vi "Filter new tree data.vi"(7 "Headers":string[](array[string]), 8 "error in":errorcluster, 9 "Root row":string[](array[string]), 10 "Child rows":string[][](array[string]), 11 "Filter":refnum<vi>) -> (0 "error out":errorcluster, 2 "Filtered child rows":string[][](array[string]), 3 "Filtered root row":string[](array[string]))   [LabVIEW 2025, in "CAN-LIN Raw Bus Capture UI.lvlib"]
uses:
  CAN-LIN Raw Bus Capture UI.lvlib
  <vilib>/Utility/error.llb/whitespace.ctl
  <vilib>/Utility/error.llb/Trim Whitespace One-Sided.vi
  Table_Filtering/Table_Filtering.lvlib
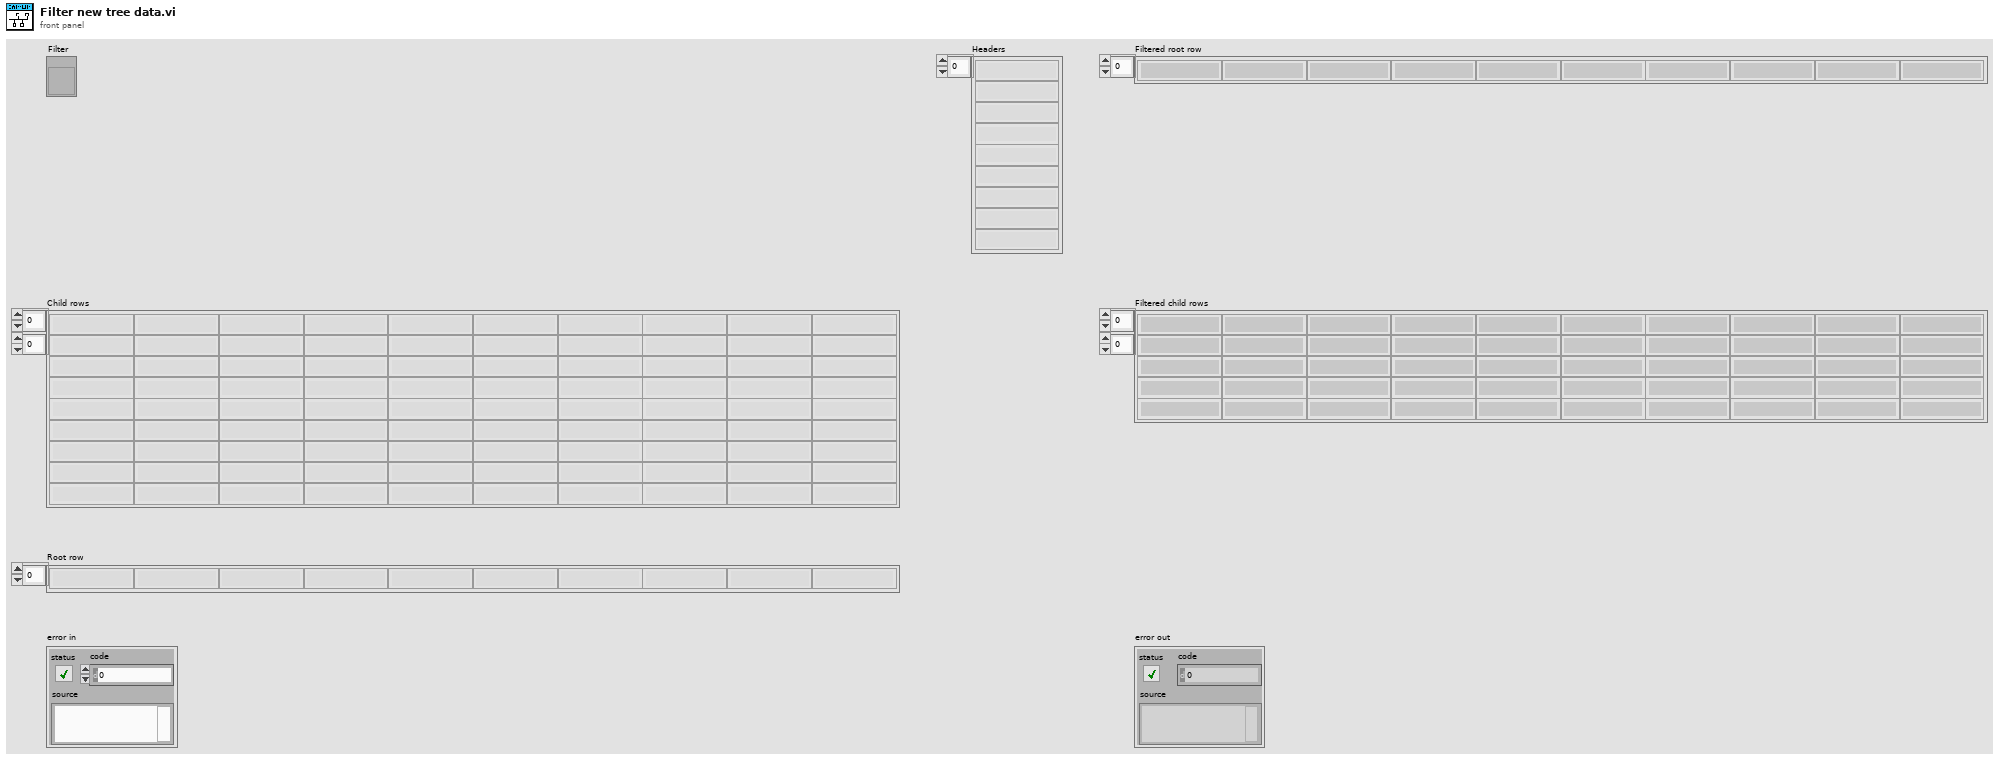
[diagram p1: front panel]
types:
  T1 = typedef "whitespace.ctl" = u16
  T2 = cluster{"FIELD":string, "OPERATOR":string, "VALUE":string}[]
  T3 = cluster{"Array":string[], "appended array":string[][]}[]
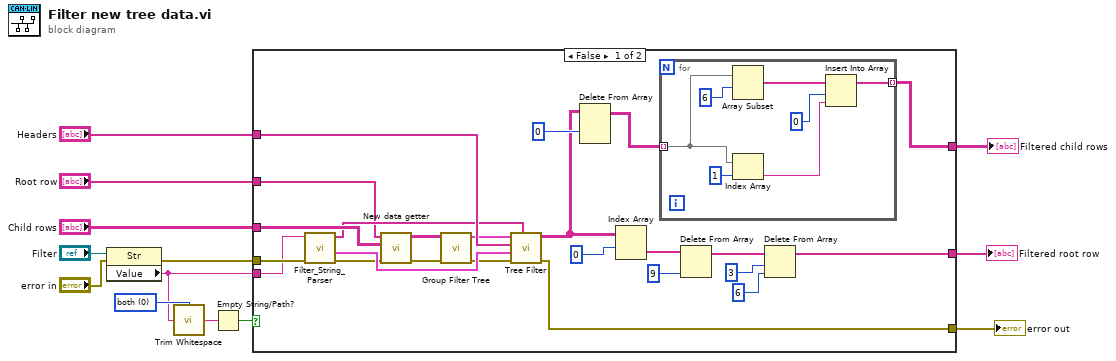
[diagram p0: block diagram]
diagram:
  w9 = T1 0 items=["both", "start of string", "end of string"] ("location (both)")
  n1 = property class="Str"(reference="Filter", error in="error in") -> (error out=w1:errorcluster, "Value"=w2:string)  [unwired: 1 out]
  n2 = call <vilib>:"Trim Whitespace.vi"("string"=w2, "location (both)"=w9) -> ("trimmed string"=w10:string)
  n3 = Empty String/Path?(string/path=w10) -> (empty?=w7:bool)
  n4 = case shown="False" w7 {
    tunnel: "Child rows" -> [w37 w45]
    tunnel: "Headers" -> [w33 _]
    tunnel: "Root row" -> [w27 w46]
    tunnel: w1 -> [w26 w47]
    tunnel: w2 -> [w25 _]
    tunnel: [w22 w47] -> w6
    tunnel: [w21 w45] -> w5
    tunnel: [w14 w46] -> w4
    frame False {
      n5 = call "Filter_String_Parser.vi"("error in"=w26, "Filter String"=w25) -> ("error constant"=w24:errorcluster, "Comparators"=w32:T2, "Boolean Connectors"=w31:string[])  [unwired: 7 in]
      n6 = call "New data getter.vi"("error in"=w24, "Child rows"=w37, "Root row"=w27) -> ("error in"=w23:errorcluster, "Root + child rows"=w28:string[][])  [unwired: 7 in]
      n7 = call "Group Filter Tree.vi"("error in"=w23, "Data in"=w28) -> ("error IO"=w30:errorcluster, "Frame groups"=w29:T3)  [unwired: 8 in]
      n8 = call "Tree Filter.vi"("Boolean Connectors"=w31, "error in"=w30, "Comparators"=w32, "Headers"=w33, "Frame groups"=w29) -> ("error out"=w22:errorcluster, "Filtered tree"=w19:string[][])  [unwired: 5 in]
      n9 = Delete From Array(array=w19, index (row)=0) -> (array with subset deleted=w18:string[][])  [unwired: 2 in, 1 out]
      n10 = Index Array(array=w19, index (row)=0) -> (element=w36:string[])  [unwired: 1 in]
      n11 = for {
        tunnel: w18 -> [w42] mode=indexing
        tunnel: [w38] -> w21 mode=indexing
        n12 = Array Subset(array=w42, index=6) -> (w43:string[])  [unwired: 1 in]
        n13 = Index Array(array=w42, index=1) -> (element=w40:string)
        n14 = Insert Into Array(array=w43, index=0, new element=w40) -> (w38:string[])
      }
      n15 = Delete From Array(array=w36, index=9) -> (array with subset deleted=w17:string[])  [unwired: 1 in, 1 out]
      n16 = Delete From Array(array=w17, length=3, index=6) -> (array with subset deleted=w14:string[])  [unwired: 1 out]
    }
    frame True {
    }
  }
  "error out" <- w6
  "Filtered child rows" <- w5
  "Filtered root row" <- w4
